vi "Military to Standard Time.vi"(8 "error in":errorcluster, 10 "Minute":i32, 11 "Hour":i32) -> (0 "error out":errorcluster, 2 "Hour":i32, 3 "Standard time":string=" 7:00 AM")   [LabVIEW 2014, in "FIRST Events API.lvlib"]
uses:
  FIRST Events API.lvlib
  <vilib>/Utility/error.llb/Error Cluster From Error Code.vi
  <vilib>/ErrorRing/Error Ring.xnode
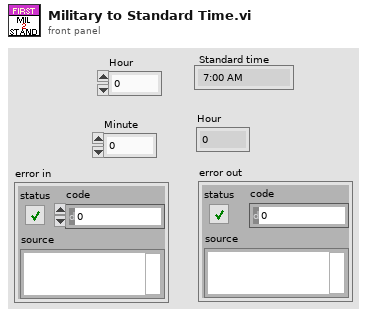
[diagram p1: front panel]
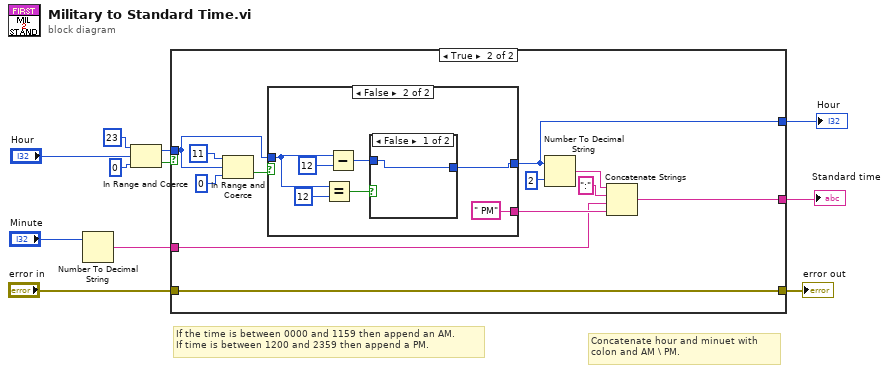
[diagram p0: block diagram]
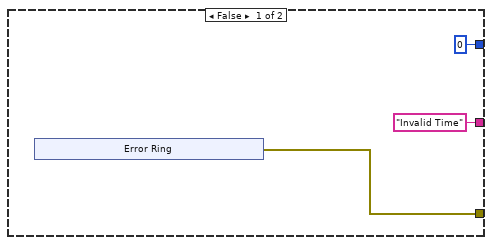
[diagram p2: hidden frame]
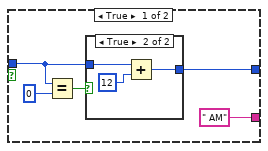
[diagram p3: hidden frame]
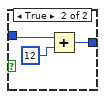
[diagram p5: hidden frame]
diagram:
  # "Concatenate hour and minuet with \ncolon and AM \\ PM."
  # "If the time is between 0000 and 1159 then append an AM.  \nIf time is between 1200 and 2359 then append a PM."
  n1 = Number To Decimal String(number="Minute") -> (decimal integer string=w5:string)  [unwired: 1 in]
  n2 = In Range and Coerce(upper limit=23, x="Hour", lower limit=0) -> (coerced(x)=w9:i32, In Range?=w8:bool)
  n3 = case shown="True" w8 {
    tunnel: w5 -> [_ w30]
    tunnel: w9 -> [_ w24]
    tunnel: [w14 w22] -> w4
    tunnel: "error in" -> [_ w22]
    tunnel: ["Invalid Time" w21] -> w2
    tunnel: [0 ("upper limit") w20] -> w1
    frame False {
      n4 = xnode "Error Ring"() -> ("error out"=w14:errorcluster)
    }
    frame True {
      n5 = In Range and Coerce(upper limit=11 ("lower limit"), x=w24, lower limit=0) -> (In Range?=w23:bool)  [unwired: 1 out]
      n6 = case shown="False" w23 {
        tunnel: [" AM" " PM"] -> w31
        tunnel: w24 -> [w35 w41]
        tunnel: [w32 w44] -> w20
        frame True {
          n7 = Equal?(x=w35, y=0) -> (x = y?=w33:bool)
          n8 = case shown="True" w33 {
            tunnel: w35 -> [w37 w40]
            tunnel: [w37 w39] -> w32
            frame False {
            }
            frame True {
              n9 = Add(x=w40, y=12 ("x+y")) -> (x+y=w39:i32)
            }
          }
        }
        frame False {
          n10 = Equal?(x=w41, y=12) -> (x = y?=w42:bool)
          n11 = Subtract(x=w41, y=12) -> (x-y=w45:i32)
          n12 = case shown="False" w42 {
            tunnel: w45 -> [w48 w51]
            tunnel: [w48 w50] -> w44
            frame False {
            }
            frame True {
              n13 = Add(x=w51, y=12 ("x+y")) -> (x+y=w50:i32)
            }
          }
        }
      }
      n14 = Number To Decimal String(number=w20, width (-)=i16 2) -> (decimal integer string=w28:string)
      n15 = Concatenate Strings(w28, ":" ("string"), w30, w31) -> (w21:string)
    }
  }
  "error out" <- w4
  "Standard time" <- w2
  "Hour" <- w1
